vi "testShouldRegisterAfterCalled.vi"(8 "error in (no error)":errorcluster, 11 "TestCase in":refnum<class "RegisterCalls.lvclass">) -> (0 "error out":errorcluster, 3 "TestCase out":refnum<class "RegisterCalls.lvclass">)   [LabVIEW 2013, in "RegisterCalls.lvclass"]
uses:
  RegisterCalls.lvclass
  Core Classes/LabSpy/Results/Been Called.vi
  <vilib>/addons/_JKI Toolkits/VI Tester/TestCase.llb/TestCase.lvclass
  Core Classes/LabSpy/LabSpy.lvclass
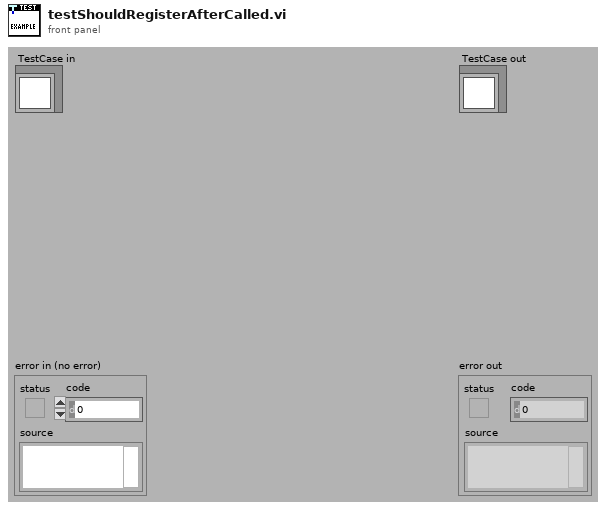
[diagram p1: front panel]
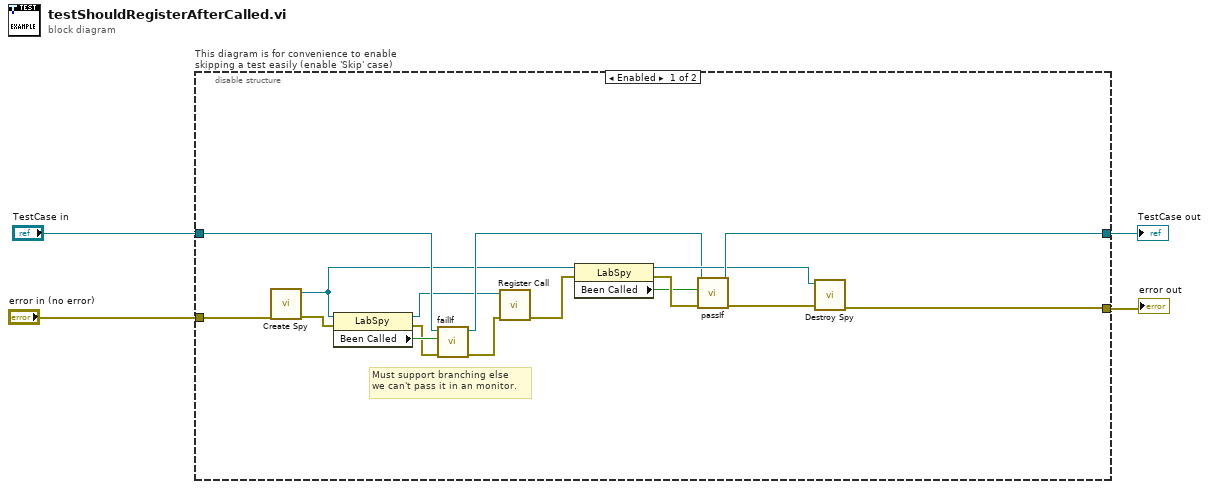
[diagram p0: block diagram]
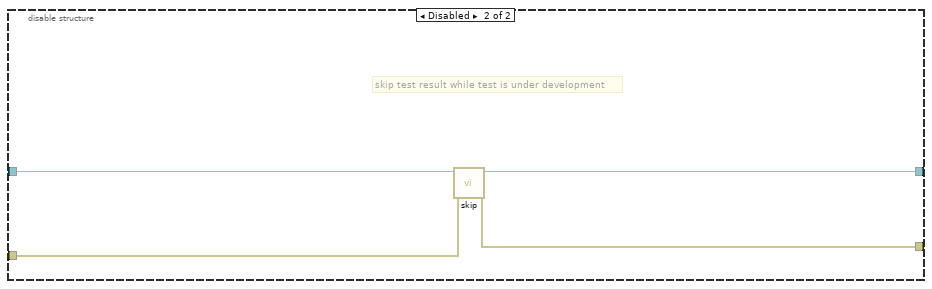
[diagram p2: hidden frame]
diagram:
  n1 = disable-structure "This diagram is for convenience to enable skipping a test easily (enable 'Skip' case)" shown="Enabled" {
    disable-tunnel: "TestCase in" -> [w10 w24]
    disable-tunnel: [w20 w22] -> w1
    disable-tunnel: [w13 w23] -> w3
    disable-tunnel: "error in (no error)" -> [w16 w21]
    frame Enabled {
      # "Must support branching else\nwe can't pass it in an monitor."
      n2 = call "Create Spy.vi"("error in (no error)"=w16) -> ("error out"=w7:errorcluster, "LabSpy Out"=w6:refnum<data-value>)  [unwired: 9 in]
      n3 = property class="LabSpy"(reference=w6, error in=w7) -> (reference out=w5:refnum<data-value>, error out=w8:errorcluster, "Been Called"=w12:bool)
      n4 = call-dynamic "failIf.vi"("error in (no error)"=w8, "fail"=w12, "TestCase in"=w10) -> ("error out"=w11:errorcluster, "TestCase out"=w9:refnum<class "RegisterCalls.lvclass">)  [unwired: 7 in]
      n5 = call "Register Call.vi"("error in (no error)"=w11, "LabSpy"=w5) -> ("error out"=w19:errorcluster)  [unwired: 8 in, 1 out]
      n6 = property class="LabSpy"(reference=w6, error in=w19) -> (reference out=w14:refnum<data-value>, error out=w18:errorcluster, "Been Called"=w17:bool)
      n7 = call-dynamic "passIf.vi"("error in (no error)"=w18, "pass"=w17, "TestCase in"=w9) -> ("error out"=w15:errorcluster, "TestCase out"=w20:refnum<class "RegisterCalls.lvclass">)  [unwired: 7 in]
      n8 = call "Destroy Spy.vi"("error in (no error)"=w15, "LabSpy"=w14) -> ("error out"=w13:errorcluster)  [unwired: 9 in]
    }
    frame Disabled {
      # "skip test result while test is under development"
      n9 = call <vilib>:"skip.vi"("error in (no error)"=w21, "TestCase in"=w24) -> ("error out"=w23:errorcluster, "TestCase out"=w22:refnum<class "RegisterCalls.lvclass">)  [unwired: 8 in]
    }
  }
  "error out" <- w3
  "TestCase out" <- w1
